vi "calculate_delta_goal.vi"(10 "Goal  Frame (World)":cluster{"X":sgl, "Y":sgl, "Theta":dbl}, 11 "Robot Heading Frame (World)":cluster{"X":sgl, "Y":sgl, "Theta":dbl}) -> (3 "Output to Goal":T2)   [LabVIEW 2016]
uses:
  <vilib>/Analysis/coordinate.llb/Angle Range (Degree).ctl
  <vilib>/Analysis/coordinate.llb/Angle Units.ctl
  <vilib>/Analysis/coordinate.llb/Wrap Angle (scalar).vi
  <vilib>/Analysis/NI_AAL_Angle.lvlib
panel:
  in  "Outpu Ref":T1
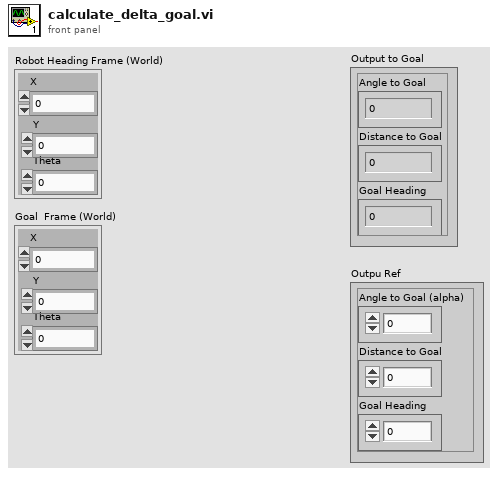
[diagram p1: front panel]
types:
  T1 = cluster{"Angle to Goal (alpha)":dbl, "Distance to Goal":sgl, "Goal Heading":sgl}
  T2 = cluster{"Angle to Goal":dbl, "Distance to Goal":sgl, "Goal Heading":sgl}
  T3 = typedef "NI_AAL_Angle.lvlib/Angle Units.ctl" = i32
  T4 = typedef "NI_AAL_Angle.lvlib/Angle Range (Degree).ctl" = u16
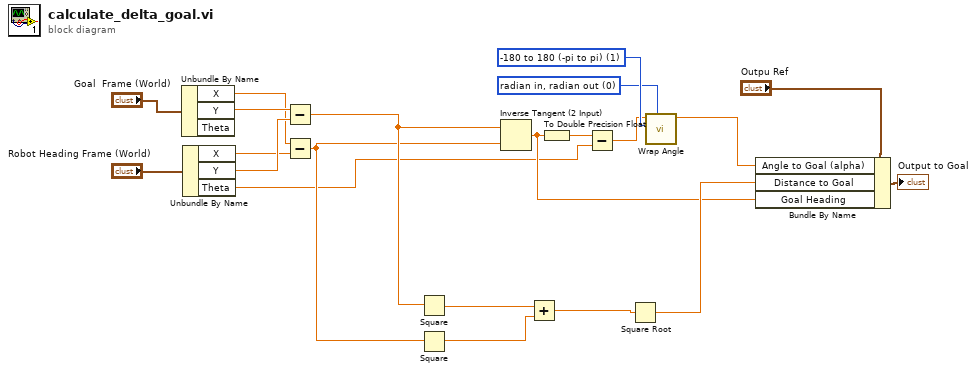
[diagram p0: block diagram]
diagram:
  w20 = T3 0 items=["radian in, radian out", "radian in, degree out", "degree in, degree out", "degree in, radian out"] ("angle units")
  w21 = T4 1 items=["none", "-180 to 180 (-pi to pi)", "0 to 360 (0 to 2pi)"] ("angle range")
  n1 = Unbundle By Name("Goal  Frame (World)") -> ("X"=w10:sgl, "Y"=w12:sgl)  [unwired: 1 out]
  n2 = Unbundle By Name("Robot Heading Frame (World)") -> ("X"=w9:sgl, "Y"=w11:sgl, "Theta"=w2:dbl)
  n3 = Subtract(x=w12, y=w11) -> (x-y=w16:sgl)
  n4 = Subtract(x=w10, y=w9) -> (x-y=w15:sgl)
  n5 = Square(x=w16) -> (x^2=w17:sgl)
  n6 = Square(x=w15) -> (x^2=w18:sgl)
  n7 = Inverse Tangent (2 Input)(1:w15, 2:w16) -> (0:w4:sgl)
  n8 = Add(x=w17, y=w18) -> (x+y=w19:sgl)
  n9 = To Double Precision Float(number=w4) -> (double precision float=w7:dbl)
  n10 = Subtract(x=w7, y=w2) -> (x-y=w8:dbl)
  n11 = Square Root(x=w19) -> (sqrt(x)=w5:sgl)
  n12 = call-poly <vilib>:"Wrap Angle.vi"("angle units"=w20, "angle range"=w21, "angle in"=w8) -> ("angle out"=w6:dbl)  [unwired: 7 in, 1 out]
  n13 = Bundle By Name(cluster="Outpu Ref", "Angle to Goal (alpha)"=w6, "Distance to Goal"=w5, "Goal Heading"=w4) -> (→"Output to Goal":T1)
